vi "FTW-JSON-Serialize.vi"(0 "JSON Object":refnum<class "FTW-JSON.lvclass">, 11 "error in":errorcluster) -> (4 "JSON Object out":refnum<class "FTW-JSON.lvclass">, 6 "JSON String (UTF-8)":string, 15 "error out":errorcluster)   [LabVIEW 2014, in "FTW-JSON.lvclass"]
uses:
  FTW-JSON.lvclass
  FTW-JSON.lvclass/FTW-JSON.ctl
panel:
  # "Inputs"
  # "Outputs"
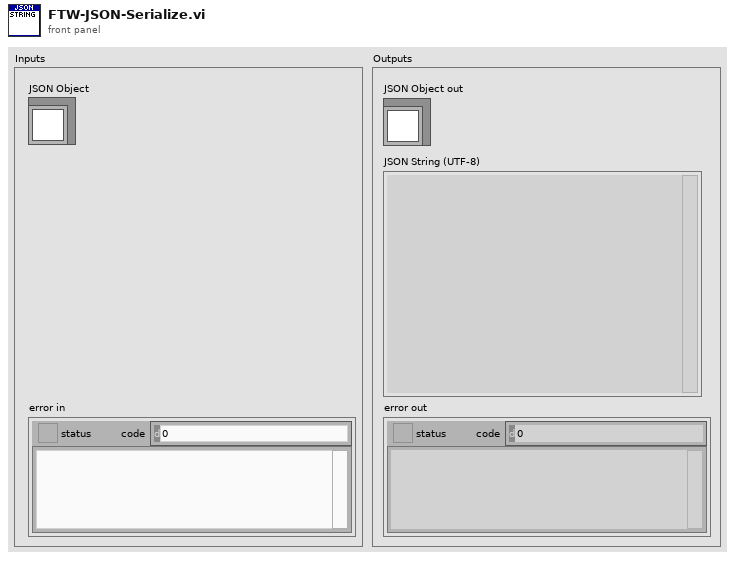
[diagram p1: front panel]
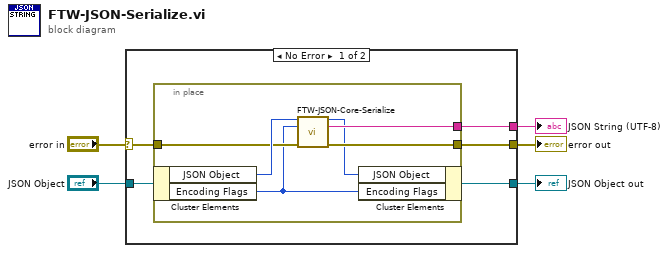
[diagram p0: block diagram]
diagram:
  n1 = case shown="No Error" "error in" {
    selector: "error in" -> [w10 w18]
    tunnel: [w9 w18] -> w5
    tunnel: [w7 w17] -> w3
    tunnel: "JSON Object" -> [w8 w17]
    tunnel: [w6 _] -> w1
    frame No Error {
      n2 = in-place {
        in-place-border: w10 -> [w15]
        in-place-border: [w13] -> w9
        in-place-border: [w12] -> w6
        n3 = in-place-cluster #1(w8) -> ("JSON Object"=w16:i64, "Encoding Flags"=w14:i64)
        n4 = call "FTW-JSON-Core-Serialize.vi"("JSON Object"=w16, "Encoding Flags"=w14, "error in"=w15) -> ("JSON Object"=w11:i64, "JSON String (UTF-8)"=w12:string, "error out"=w13:errorcluster)  [unwired: 10 in]
        n5 = in-place-cluster #1("JSON Object"=w11, "Encoding Flags"=w14) -> (w7:refnum<class "FTW-JSON.lvclass">)
      }
    }
    frame Error {
    }
  }
  "error out" <- w5
  "JSON Object out" <- w3
  "JSON String (UTF-8)" <- w1
